vi "12a Find short path.vi"(9 "End Point>>":T1, 10 "Start Point":T1, 11 "Field Elevation":u8[][](array[numeric])) -> (1 "Array Out":i32[][](array[numeric]), 3 "Enpoint Value Out":i32, 5 "Map Out":map{T1, i32}(c390))   [LabVIEW 2020]
uses:
  Cluster Point.ctl
  654511ec-6e94-42fe-afcb-f29a0aa8742f.vi
  <vilib>/Comparison/Less/Less Functor/Less Functor.lvclass
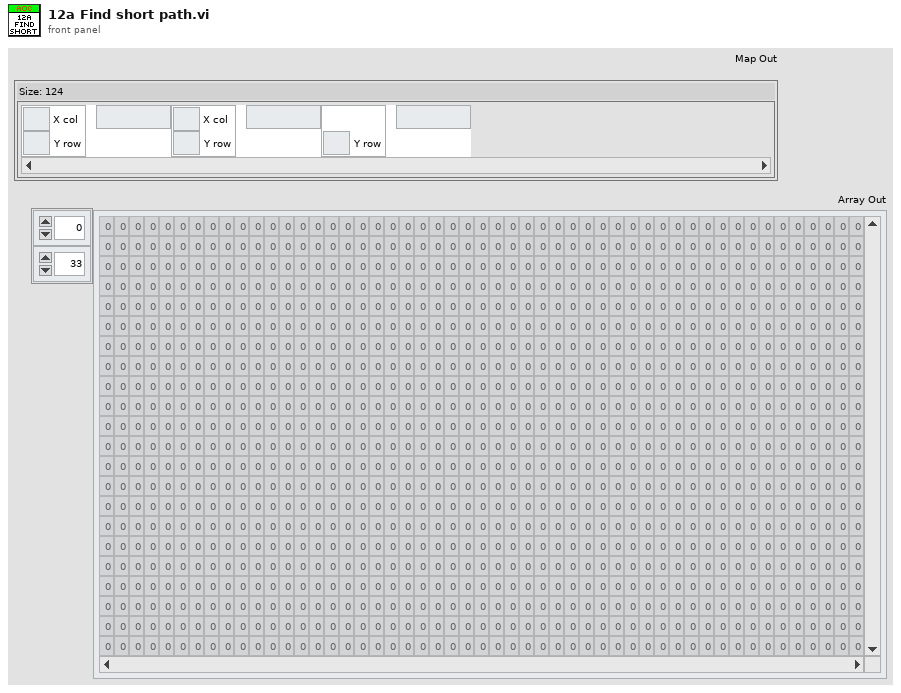
[diagram p1: front panel]
types:
  T1 = typedef "Cluster Point.ctl" = cluster{"X col":i32, "Y row":i32}
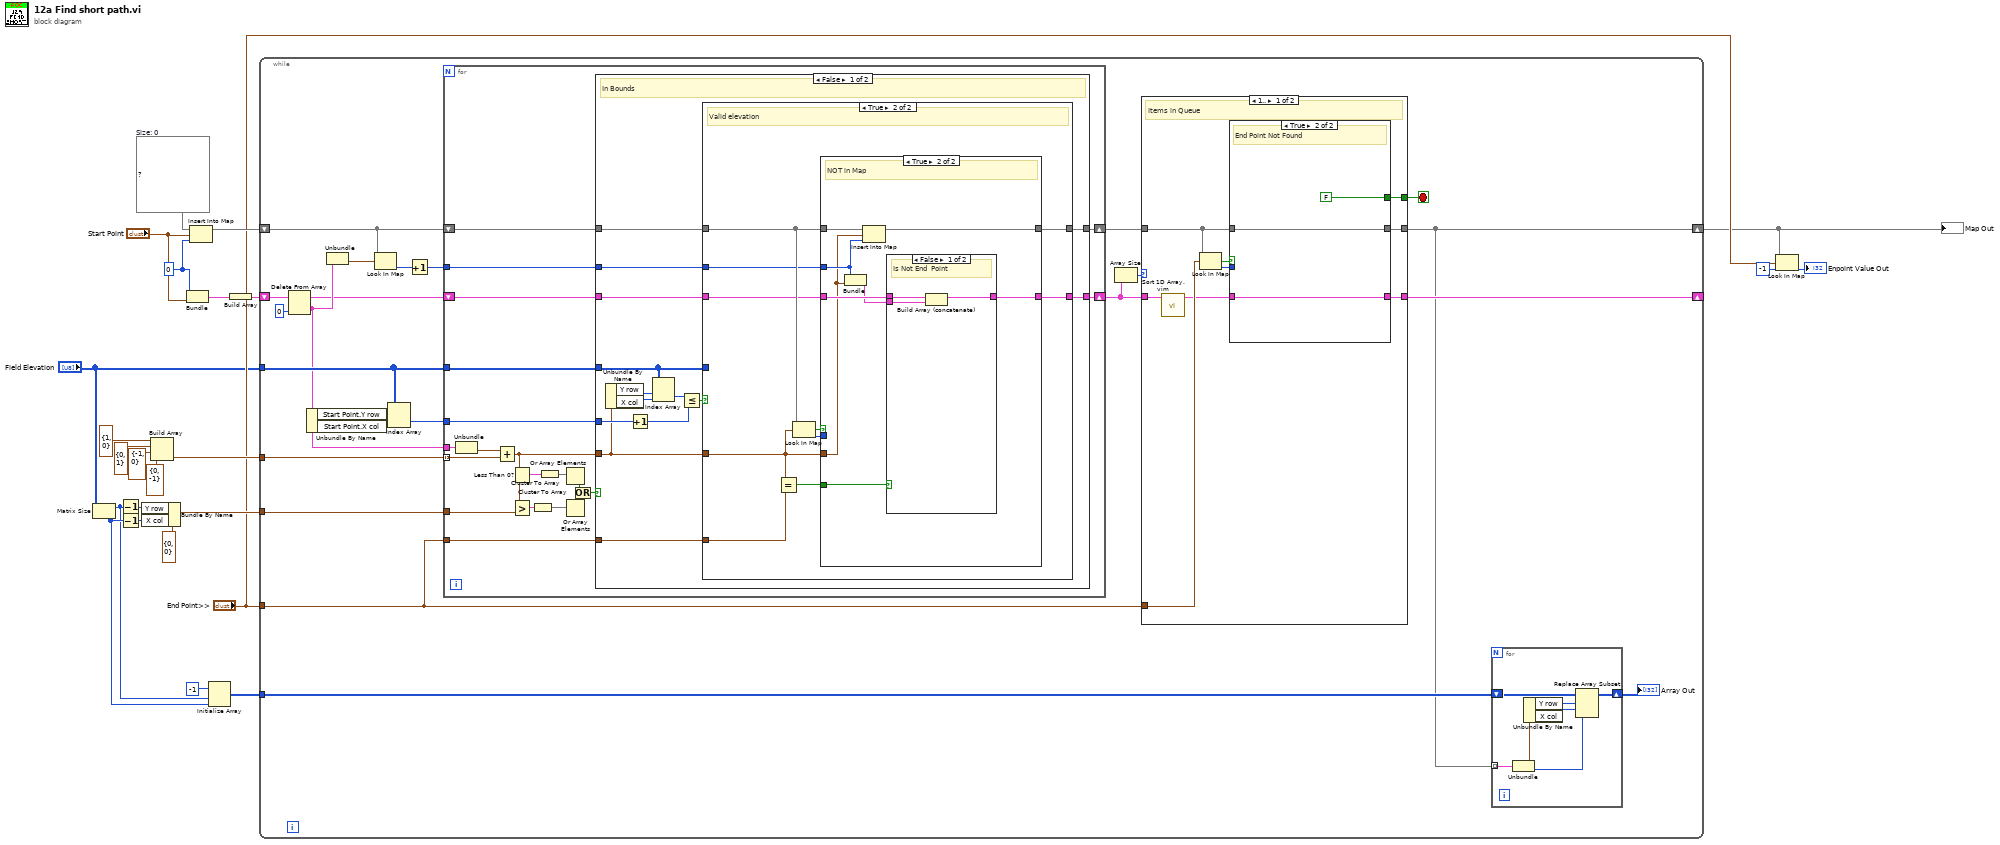
[diagram p0: block diagram]
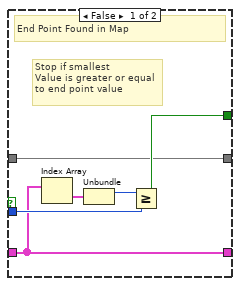
[diagram p2: hidden frame]
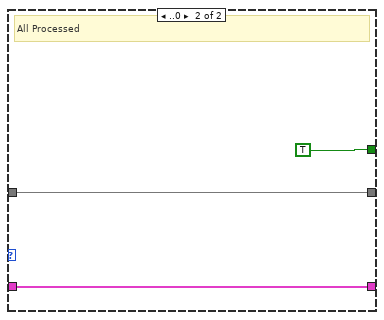
[diagram p3: hidden frame]
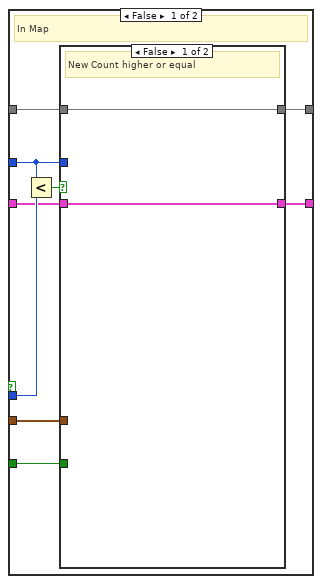
[diagram p5: hidden frame]
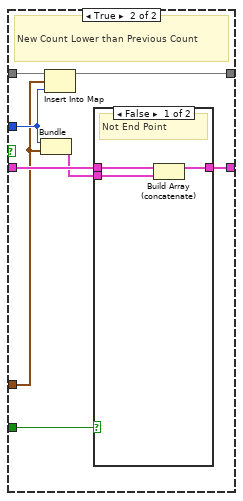
[diagram p6: hidden frame]
diagram:
  w18 = 0 ("value")
  w15 = map{T1, i32} {}  # Size: 0
  n1 = Matrix Size(0:"Field Elevation") -> (1:w22:i32, 2:w23:i32)
  n2 = Decrement(x=w22) -> (x-1=w13:i32)
  n3 = Decrement(x=w23) -> (x-1=w14:i32)
  n4 = Bundle By Name(cluster=T1 {"X col"=0, "Y row"=0} ("unsigned byte array"), "Y row"=w13, "X col"=w14) -> (w12:T1)
  n5 = Build Array(T1 {"X col"=1, "Y row"=0} ("unsigned byte array"), T1 {"X col"=0, "Y row"=1} ("unsigned byte array"), T1 {"X col"=-1, "Y row"=0} ("unsigned byte array"), T1 {"X col"=0, "Y row"=-1} ("unsigned byte array")) -> (w7:T1[])
  n6 = Bundle("value"=w18, "Start Point"="Start Point") -> (w20:cluster{"value":i32, "Start Point":T1})  [unwired: 1 in]
  n7 = Insert Into Map(map in=w15, key="Start Point", value=w18) -> (map out=w16:map{T1, i32})  [unwired: 2 out]
  n8 = Initialize Array(-1, w22, w23) -> (w24:i32[][])
  n9 = Build Array(w20) -> (w17:cluster{"value":i32, "Start Point":T1}[])
  n10 = while {
    tunnel: w7 -> [w47]
    tunnel: "Field Elevation" -> [w41]
    tunnel: w12 -> [w46]
    tunnel: "End Point>>" -> [w30]
    shift-right: [w26] -> w3
    shift-left: w16 -> [w28]
    shift-right: [w34] -> _
    shift-left: w17 -> [w39]
    tunnel: w24 -> [w27]
    stop <- w32 stop-if-true
    n11 = Delete From Array(array=w39, index=0) -> (deleted portion=w38:cluster{"value":i32, "Start Point":T1}, array with subset deleted=w37:cluster{"value":i32, "Start Point":T1}[])  [unwired: 1 in]
    n12 = Unbundle By Name(w38) -> ("Start Point.Y row"=w43:i32, "Start Point.X col"=w42:i32)
    n13 = Unbundle(w38) -> ("Start Point"=w31:T1)  [unwired: 1 out]
    n14 = Look In Map(map=w28, key=w31) -> (value=w45:i32)  [unwired: 1 in, 1 out]
    n15 = Index Array(array=w41, index (row)=w43, index (col)=w42) -> (element=w40:u8)
    n16 = Increment(x=w45) -> (x+1=w44:i32)
    n17 = for {
      tunnel: w47 -> [w95] mode=indexing
      tunnel: w46 -> [w78]
      tunnel: w41 -> [w86]
      tunnel: w38 -> [w91]
      shift-right: [w80] -> w33
      shift-left: w28 -> [w82]
      tunnel: w44 -> [w83]
      tunnel: w40 -> [w84]
      shift-right: [w79] -> w35
      shift-left: w37 -> [w81]
      tunnel: w30 -> [w76]
      n18 = Unbundle(w91) -> ("Start Point"=w77:T1)  [unwired: 1 out]
      n19 = Add(x=w77, y=w95) -> (x+y=w85:T1)
      n20 = Less Than 0?(x=w85) -> (x < 0?=w90:cluster{"X col":bool, "Y row":bool})
      n21 = Greater?(x=w85, y=w78) -> (0:w88:cluster{"X col":bool, "Y row":bool})
      n22 = Cluster To Array(cluster=w88) -> (array=w87:bool[])
      n23 = Cluster To Array(cluster=w90) -> (array=w89:bool[])
      n24 = Or Array Elements(Boolean array=w89) -> (logical OR=w93:bool)
      n25 = Or Array Elements(Boolean array=w87) -> (logical OR=w94:bool)
      n26 = Or(x=w93, y=w94) -> (x .or. y?=w92:bool)
      n27 = case shown="False" w92 {
        tunnel: w86 -> [w103 _]
        tunnel: w85 -> [w101 _]
        tunnel: w84 -> [w107 _]
        tunnel: w83 -> [w102 _]
        tunnel: w82 -> [w100 w158]
        tunnel: w81 -> [w99 w157]
        tunnel: [w98 w158] -> w80
        tunnel: [w97 w157] -> w79
        tunnel: w76 -> [w96 _]
        frame False {
          # "In Bounds"
          n28 = Unbundle By Name(w101) -> ("Y row"=w108:i32, "X col"=w109:i32)
          n29 = Increment(x=w107) -> (x+1=w105:u8)
          n30 = Index Array(array=w103, index (row)=w108, index (col)=w109) -> (element=w106:u8)
          n31 = Less Or Equal?(x=w106, y=w105) -> (x <= y?=w104:bool)
          n32 = case shown="True" w104 {
            tunnel: w103 -> [_ _]
            tunnel: w102 -> [_ w120]
            tunnel: w101 -> [_ w113]
            tunnel: w100 -> [w111 w121]
            tunnel: w99 -> [w110 w119]
            tunnel: [w111 w118] -> w98
            tunnel: [w110 w117] -> w97
            tunnel: w96 -> [_ w114]
            frame False {
              # "Point too High"
            }
            frame True {
              # "Valid elevation"
              n33 = Equal?(x=w113, y=w114) -> (x = y?=w112:bool)
              n34 = Look In Map(map=w121, key=w113) -> (key not found?=w116:bool, value=w115:i32)  [unwired: 1 in]
              n35 = case shown="True" w116 {
                tunnel: w115 -> [w130 _]
                tunnel: w121 -> [w128 w152]
                tunnel: w113 -> [w124 w147]
                tunnel: w120 -> [w125 w148]
                tunnel: w119 -> [w126 w150]
                tunnel: [w127 w151] -> w118
                tunnel: [w123 w149] -> w117
                tunnel: w112 -> [w122 w145]
                frame False {
                  # "In Map"
                  n36 = Less?(x=w125, y=w130) -> (x < y?=w129:bool)
                  n37 = case shown="False" w129 {
                    tunnel: w128 -> [w132 w140]
                    tunnel: [w132 w139] -> w127
                    tunnel: w126 -> [w131 w138]
                    tunnel: w125 -> [_ w136]
                    tunnel: w124 -> [_ w134]
                    tunnel: [w131 w137] -> w123
                    tunnel: w122 -> [_ w133]
                    frame False {
                      # "New Count higher or equal"
                    }
                    frame True {
                      # "New Count Lower than Previous Count"
                      n38 = Bundle(w136, "Start Point"=w134) -> (w135:cluster{i32, "Start Point":T1})  [unwired: 1 in]
                      n39 = Insert Into Map(map in=w140, key=w134, value=w136) -> (map out=w139:map{T1, i32})  [unwired: 2 out]
                      n40 = case shown="False" w133 {
                        tunnel: w138 -> [w143 w144]
                        tunnel: [w142 w144] -> w137
                        tunnel: w135 -> [w141 _]
                        frame False {
                          # "Not End Point"
                          n41 = Build Array (concatenate)(w143, w141) -> (w142:cluster{"value":i32, "Start Point":T1}[])
                        }
                        frame True {
                          # "Is End Point"
                        }
                      }
                    }
                  }
                }
                frame True {
                  # "NOT in Map"
                  n42 = Bundle(w148, "Start Point"=w147) -> (w146:cluster{i32, "Start Point":T1})  [unwired: 1 in]
                  n43 = Insert Into Map(map in=w152, key=w147, value=w148) -> (map out=w151:map{T1, i32})  [unwired: 2 out]
                  n44 = case shown="False" w145 {
                    tunnel: w150 -> [w155 w156]
                    tunnel: [w154 w156] -> w149
                    tunnel: w146 -> [w153 _]
                    frame False {
                      # "Is Not End  Point"
                      n45 = Build Array (concatenate)(w155, w153) -> (w154:cluster{"value":i32, "Start Point":T1}[])
                    }
                    frame True {
                      # "Is End Point"
                    }
                  }
                }
              }
            }
          }
        }
        frame True {
          # "Out Of Bounds"
        }
      }
    }
    n46 = Array Size(array=w35) -> (size(s)=w36:i32)
    n47 = case shown="1.." w36 {
      tunnel: w35 -> [w55 w75]
      tunnel: [w57 w75] -> w34
      tunnel: w33 -> [w61 w74]
      tunnel: [w59 w74] -> w26
      tunnel: [w58 TRUE] -> w32
      tunnel: w30 -> [w63 _]
      frame 1.. {
        # "Items in Queue"
        n48 = call "Sort 1D Array.vim"("unsorted array"=w55) -> ("sorted array"=w56:cluster{"value":i32, "Start Point":T1}[])  [unwired: 10 in]
        n49 = Look In Map(map=w61, key=w63) -> (key not found?=w62:bool, value=w60:i32)  [unwired: 1 in]
        n50 = case shown="True" w62 {
          tunnel: w61 -> [w65 w72]
          tunnel: w60 -> [w67 _]
          tunnel: [w65 w72] -> w59
          tunnel: [w66 FALSE] -> w58
          tunnel: w56 -> [w64 w70]
          tunnel: [w64 w70] -> w57
          frame False {
            # "Stop if smallest\nValue is greater or equal\nto end point value"
            # "End Point Found in Map"
            n51 = Index Array(array=w64) -> (element=w69:cluster{"value":i32, "Start Point":T1})  [unwired: 1 in]
            n52 = Unbundle(w69) -> ("value"=w68:i32)  [unwired: 1 out]
            n53 = Greater Or Equal?(x=w68, y=w67) -> (x >= y?=w66:bool)
          }
          frame True {
            # "End Point Not Found"
          }
        }
      }
      frame ..0 {
        # "All Processed"
      }
    }
    n54 = for {
      tunnel: w26 -> [w54] mode=indexing
      shift-right: [w52] -> w25
      shift-left: w27 -> [w53]
      n55 = Unbundle(w54) -> ("Point"=w51:T1, "min step"=w48:i32)
      n56 = Unbundle By Name(w51) -> ("Y row"=w50:i32, "X col"=w49:i32)
      n57 = Replace Array Subset(array=w53, new element=w48, index (row)=w50, index (col)=w49) -> (w52:i32[][])
    }
    "Array Out" <- w25
  }
  "Map Out" <- w3
  n58 = Look In Map(map=w3, key="End Point>>", default value=-1) -> (value=→"Enpoint Value Out":i32)  [unwired: 1 out]
